vi "get cal file path.vi"(10 "Glass Motor?":bool, 11 "Part Type":string) -> (3 "appended path":path)   [LabVIEW 2018]
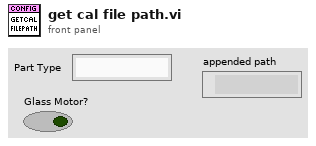
[diagram p1: front panel]
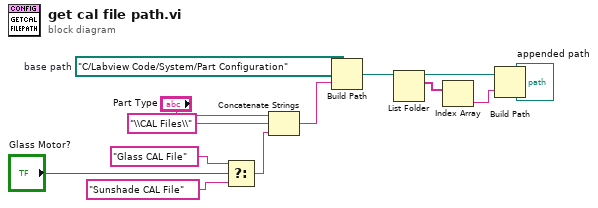
[diagram p0: block diagram]
diagram:
  w9 = path "C:/Labview Code/System/Part Configuration"  # base path
  n1 = Select(t="Glass CAL File", s="Glass Motor?", f="Sunshade CAL File") -> (s? t:f=w3:string)
  n2 = Concatenate Strings("Part Type", "\\CAL Files\\", w3) -> (w4:string)
  n3 = Build Path(base path=w9, name or relative path=w4) -> (appended path=w10:path)
  n4 = List Folder(path=w10) -> (path out=w11:path, filenames=w12:string[])  [unwired: 3 in, 2 out]
  n5 = Index Array(array=w12) -> (element=w13:string)  [unwired: 1 in]
  n6 = Build Path(base path=w11, name or relative path=w13) -> (appended path=→"appended path":path)
